vi "LWXPS_PositionerCorrectorDamperFilterGet.vi"(0 "XPS Reference IN":refnum<k24>, 7 "Positioner Name":string, 11 "LabVIEW error IN":errorcluster) -> (3 "XPS Reference OUT":refnum<k24>, 4 "Returned error code":i32, 6 "Damping Factor":dbl, 8 "Filter Gain":dbl, 10 "Cut Off Frequency":dbl, 14 "LabVIEW error OUT":errorcluster, 15 "XPS Error String":string)   [LabVIEW 2014]
uses:
  D:/XPSQ8_LabView_Library/Development/Source/Dll/Newport.XPS.CommandInterface.dll
  Dll/Newport.XPS.CommandInterface.dll
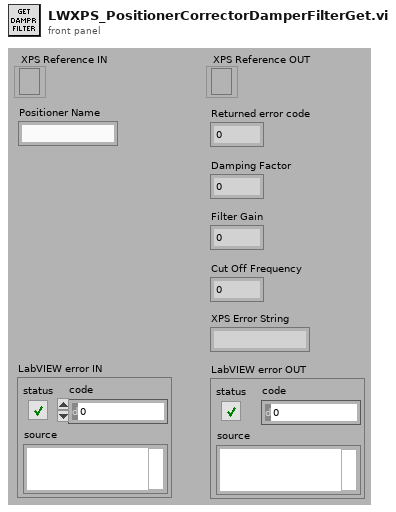
[diagram p1: front panel]
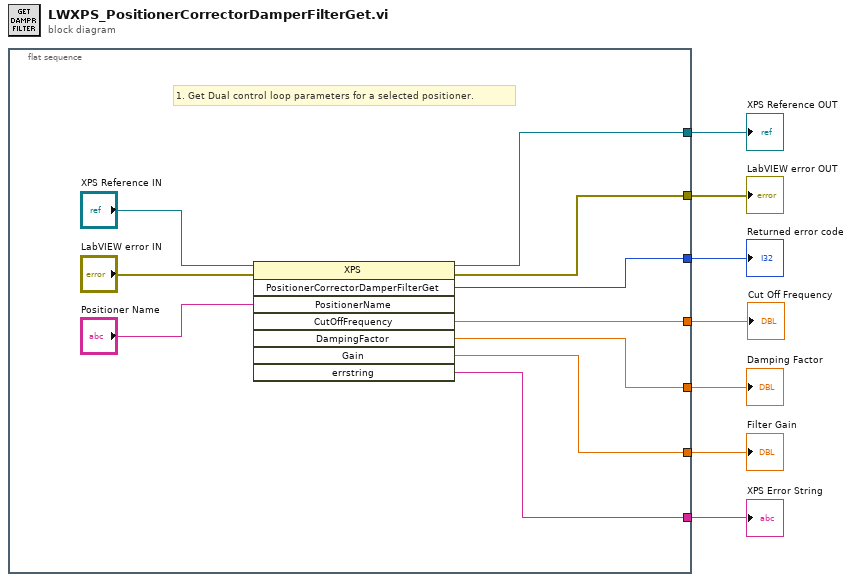
[diagram p0: block diagram]
diagram:
  n1 = flat-sequence {
    tunnel: [w15] -> w7
    tunnel: [w10] -> w6
    tunnel: [w16] -> w5
    tunnel: [w8] -> w4
    tunnel: [w12] -> w3
    tunnel: [w11] -> w1
    tunnel: [w9] -> w2
    frame #0 {
      # "1. Get Dual control loop parameters for a selected positioner."
      n2 = invoke class="XPS" method="PositionerCorrectorDamperFilterGet"(reference="XPS Reference IN", error in="LabVIEW error IN", "PositionerName"="Positioner Name") -> (reference out=w15:refnum<k24>, error out=w10:errorcluster, "PositionerCorrectorDamperFilterGet"=w16:i32, "CutOffFrequency"=w9:dbl, "DampingFactor"=w8:dbl, "Gain"=w12:dbl, "errstring"=w11:string)  [unwired: 5 in, 1 out]
    }
  }
  "XPS Error String" <- w1
  "XPS Reference OUT" <- w7
  "LabVIEW error OUT" <- w6
  "Returned error code" <- w5
  "Damping Factor" <- w4
  "Filter Gain" <- w3
  "Cut Off Frequency" <- w2
